vi "Format Event.vi"(0 "StatD Interface in":refnum<class "StatD Interface.lvclass">, 1 "Tags":string[](array[string]), 3 "Tag Values":string[](array[string]), 5 "Event Title":string, 7 "Event Text":string, 9 "Event Type":T2, 11 "error in (no error)":errorcluster, 12 "Priority (normal)":T1=enum."normal", 13 "Aggregation Key (none)":string) -> (4 "StatD Interface out":refnum<class "StatD Interface.lvclass">, 6 "Packet":string, 15 "error out":errorcluster)   [LabVIEW 2011, in "StatD Interface.lvclass"]
doc: "Formats a packet to send an event to the statd collector."
uses:
  StatD Interface.lvclass
  Controls/Event Types.ctl
  Controls/Priorities.ctl
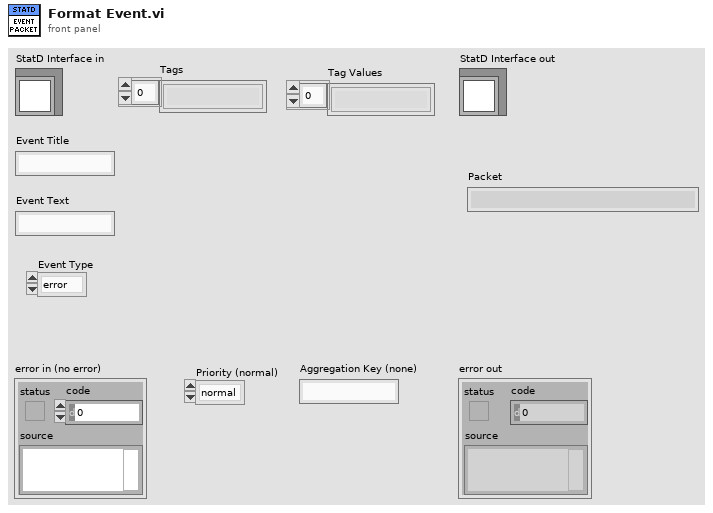
[diagram p1: front panel]
types:
  T1 = typedef "StatD Interface.lvclass/Priorities.ctl" = enum16{"low", "normal"}
  T2 = typedef "StatD Interface.lvclass/Event Types.ctl" = enum16{"error", "warning", "info", "success"}
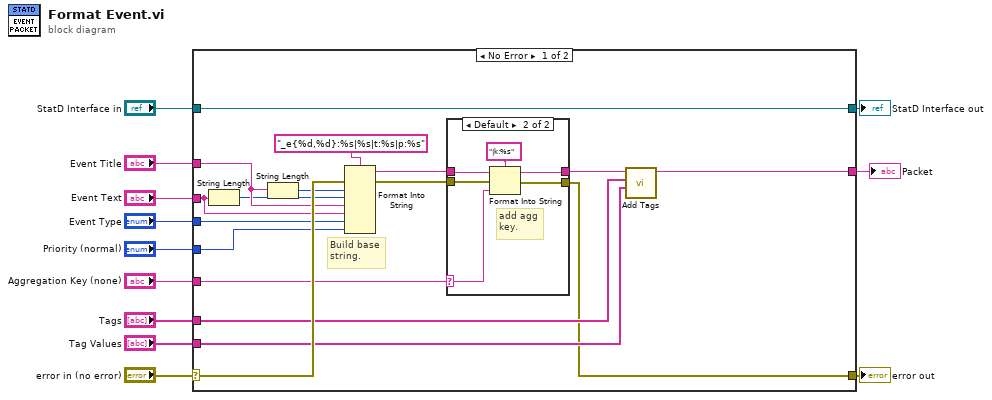
[diagram p0: block diagram]
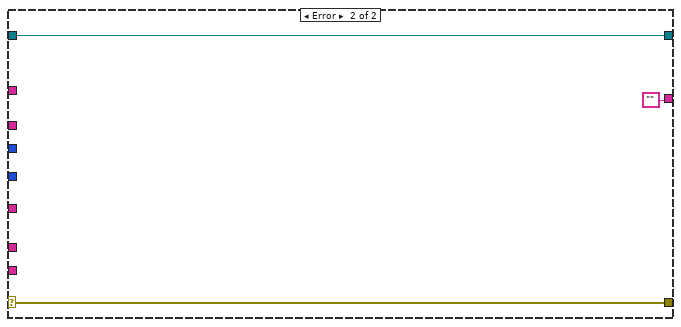
[diagram p3: hidden frame]
diagram:
  n1 = case shown="No Error" "error in (no error)" {
    selector: "error in (no error)" -> [w27 w40]
    tunnel: [w13 w40] -> w11
    tunnel: [w29 w39] -> w9
    tunnel: "StatD Interface in" -> [w29 w39]
    tunnel: "Event Title" -> [w22 _]
    tunnel: "Tags" -> [w26 _]
    tunnel: "Tag Values" -> [w25 _]
    tunnel: [w24 ""] -> w5
    tunnel: "Event Text" -> [w20 _]
    tunnel: "Event Type" -> [w19 _]
    tunnel: "Priority (normal)" -> [w18 _]
    tunnel: "Aggregation Key (none)" -> [w17 _]
    frame No Error {
      # "Build base\nstring."
      n2 = String Length(string=w20) -> (length=w21:i32)
      n3 = String Length(string=w22) -> (length=w23:i32)
      n4 = Format Into String(format string="_e{%d,%d}:%s|%s|t:%s|p:%s", error in=w27, w23, w21, w22, w20, w19, w18) -> (resulting string=w15:string, error out=w14:errorcluster)  [unwired: 1 in]
      n5 = case shown="Default" w17 {
        selector: w17 -> [_ w34]
        tunnel: [w31 w36] -> w16
        tunnel: w15 -> [w31 w37]
        tunnel: w14 -> [w30 w33]
        tunnel: [w30 w32] -> w13
        frame "" {
          # "no agg key."
        }
        frame Default {
          # "add agg\nkey."
          n6 = Format Into String(format string="|k:%s", initial string=w37, error in=w33, w34) -> (resulting string=w36:string, error out=w32:errorcluster)
        }
      }
      n7 = call "Add Tags.vi"("Tag Values"=w25, "Tags"=w26, "Packet in"=w16) -> ("Packet out"=w24:string)  [unwired: 8 in]
    }
    frame Error {
    }
  }
  "error out" <- w11
  "StatD Interface out" <- w9
  "Packet" <- w5
